vi "CallBack_MouseWheel.vi"(4 "Data":T1, 5 "Event Data":cluster{"sender":refnum<k24>, "e":refnum<k24>}, 6 "Control Ref":refnum<k24>, 7 "Event Common Data":T2) -> ()   [LabVIEW 2020, in "LcPictureBox.lvclass"]
uses:
  LcPictureBox.lvclass
  CallBacks/MouseWheelInfo.ctl
  System.Windows.Forms
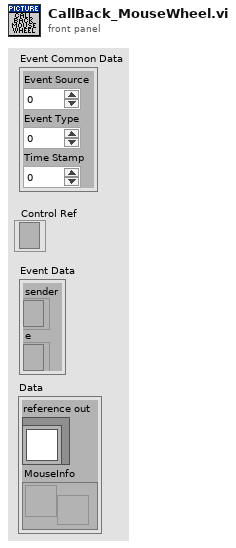
[diagram p1: front panel]
types:
  T1 = cluster{"reference out":refnum<class "LcPictureBox.lvclass">, "MouseInfo":refnum<user-event>}
  T2 = cluster{"Event Source":i32, "Event Type":u32, "Time Stamp":u32}
  T3 = typedef "LcPictureBox.lvclass/MouseWheelInfo.ctl" = cluster{"X":i32, "Y":i32, "Button":i32, "Delta":i32, "X(raw)":i32, "Y(raw)":i32}
  T4 = typedef "LcPictureBox.lvclass/ObjectAttributes.ctl" = cluster{"PictureBox":refnum<k24>, "ImageSize":cluster{"Width":i32, "Height":i32}, "PenMemory":map{cluster{"Alpha(100%)":dbl, "Color(Black)":u32, "Pen(Width=1, Solid)":T5}, refnum<k24>}, "GraphicsRef":refnum<k24>, "BrushMemory":map{cluster{"Alpha(100%)":dbl, "Color(Black)":u32}, refnum<k24>}, "Images":refnum<k24>[], "ImageIndex":i32, "BgColor(None)":u32, "LoadedImages":map{string, cluster{"ImageOut":refnum<k24>, "ImageSize":cluster{"Width":i32, "Height":i32}}}, "ColorsMemory":map{cluster{"Alpha(100%)":dbl, "Color(Black)":u32}, refnum<k24>}, "CacheSize":i32, "PictureBoxActiveXReference":refnum<vi>, "Scale":sgl, "Offset":cluster{"x":sgl, "y":sgl}, "zoom_center":cluster{"X":i32, "Y":i32}, "ImagesCreated":refnum<k24>[]}
  T5 = typedef "LcPictureBox.lvclass/Pen.ctl" = cluster{"Width":u16, "Style":enum32{"Solid", "Dash", "Dot", "DashDot", "DashDotDot"}}
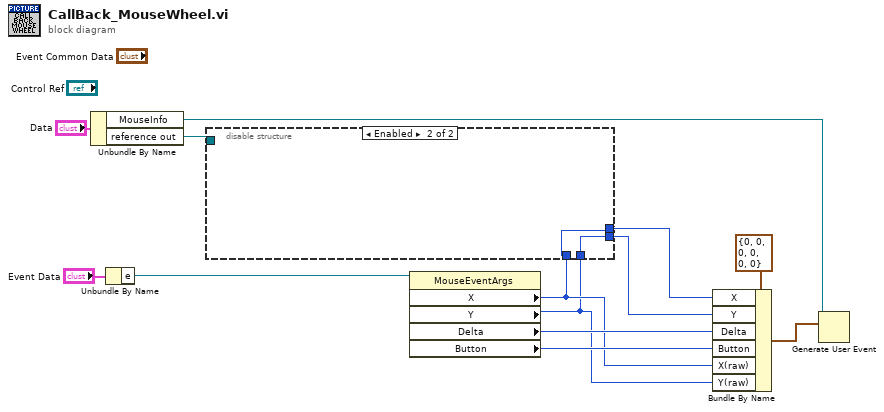
[diagram p0: block diagram]
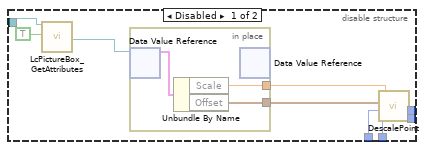
[diagram p2: hidden frame]
diagram:
  n1 = Unbundle By Name("Data") -> ("MouseInfo"=w4:refnum<user-event>, "reference out"=w5:refnum<class "LcPictureBox.lvclass">)
  n2 = Unbundle By Name("Event Data") -> ("e"=w13:refnum<k24>)
  n3 = property class="MouseEventArgs"(reference=w13) -> ("X"=w2:i32, "Y"=w1:i32, "Delta"=w12:i32, "Button"=w9:i32)  [unwired: 1 in, 2 out]
  n4 = disable-structure shown="Enabled" {
    disable-tunnel: [w22 w27] -> w8
    disable-tunnel: [w21 w26] -> w7
    disable-tunnel: w5 -> [w19 _]
    disable-tunnel: w2 -> [w15 w27]
    disable-tunnel: w1 -> [w14 w26]
    frame Disabled {
      n5 = call "LcPictureBox_GetAttributes.vi"("reference in"=w19, "OnlyGetDvrReference(False)"=TRUE) -> ("DataRef"=w18:refnum<data-value>)  [unwired: 14 in, 3 out]
      n6 = in-place {
        in-place-border: [w24] -> w16
        in-place-border: [w23] -> w17
        n7 = in-place-dvr #1(w18) -> (w25:T4)  [unwired: 1 out]
        n8 = Unbundle By Name(w25) -> ("Scale"=w23:sgl, "Offset"=w24:cluster{"x":sgl, "y":sgl})
        n9 = in-place-dvr #1() -> ()  [unwired: 1 in, 2 out]
      }
      n10 = call "DescalePoint.vi"("Y"=w14, "X"=w15, "Offset"=w16, "Scale"=w17) -> ("Y-Out"=w21:sgl, "X-Out"=w22:sgl)  [unwired: 6 in]
    }
    frame Enabled {
    }
  }
  n11 = Bundle By Name(cluster=T3 {"X"=0, "Y"=0, "Button"=0, "Delta"=0, "X(raw)"=0, "Y(raw)"=0} ("MouseInfo"), "X"=w8, "Y"=w7, "Delta"=w12, "Button"=w9, "X(raw)"=w2, "Y(raw)"=w1) -> (w3:T3)
  n12 = Generate User Event(user event=w4, event data cluster=w3) -> ()  [unwired: 2 in, 2 out]
